vi "Parse String Fields.vi"(8 "Separator":string=":", 11 "String":string) -> (0 "Number of fields":u32, 3 "Fields":string[](array[string]))   [LabVIEW 2020]
doc: "Returns an array of Fields parsed out of String. Fields are separated by the string Separator (default \":\")."
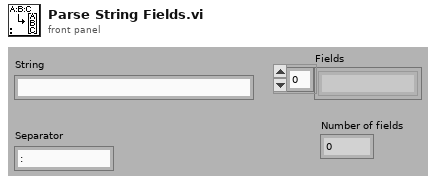
[diagram p1: front panel]
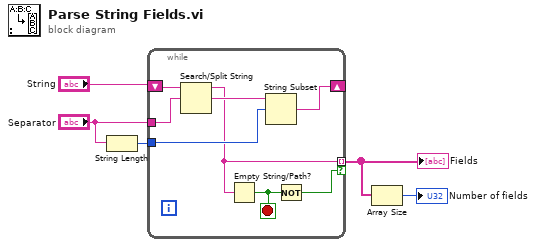
[diagram p0: block diagram]
diagram:
  n1 = String Length(string="Separator") -> (length=w2:i32)
  n2 = while {
    shift-right: [w11] -> _
    shift-left: "String" -> [w13]
    tunnel: "Separator" -> [w10]
    tunnel: w2 -> [w9]
    tunnel: [w8] -> w1 mode=indexing if=w6
    stop <- w7 stop-if-true
    n3 = Search/Split String(string=w13, search string/char (-)=w10) -> (substring before match=w8:string, match + rest of string=w12:string)  [unwired: 1 in, 1 out]
    n4 = Empty String/Path?(string/path=w8) -> (empty?=w7:bool)
    n5 = String Subset(string=w12, offset (0)=w9) -> (substring=w11:string)  [unwired: 1 in]
    n6 = Not(x=w7) -> (.not. x?=w6:bool)
  }
  "Fields" <- w1
  n7 = Array Size(array=w1) -> (size(s)=→"Number of fields":i32)
